vi "Estimate Test Coverage - Main UI - .vi"(10 "Test Path (Tests folder -- including _framework)":path, 11 "Source Path (lvproj, lvclass, vi)":path) -> ()   [LabVIEW 2009]
uses:
  Graphical Test Runner/Graphical Test Runner Support/EstimationResults--Cluster.ctl
  Graphical Test Runner/Graphical Test Runner Support/ScanOptions--Cluster.ctl
  Graphical Test Runner/Graphical Test Runner Support/GraphicalTestRunner.lvlib
panel:
  in  "Estimation Tabs":enum32{"Graphs", "Metrics", "Files", "Setup"}(tab)
  out "Bar Graph":picture caption="Percentage of Test Gaps By Folder"
  in  "Coverage Graph":T1(ring)
  out "Percent Coverage":u8
  out "Total Test VIs":i32
  out "Untested Project VIs":i32
  out "Pass":bool
  in  "Files without coverage":i32(listbox)
  in  "Minimum Coverage (%)":dbl
  in  "Ignore reuse libraries":bool=TRUE
  in  "Ignore non VIs":bool=TRUE
  in  "Abort":bool
  in  "Estimate":bool
  in  "Exit":bool
  # "Estimate Test Coverage"
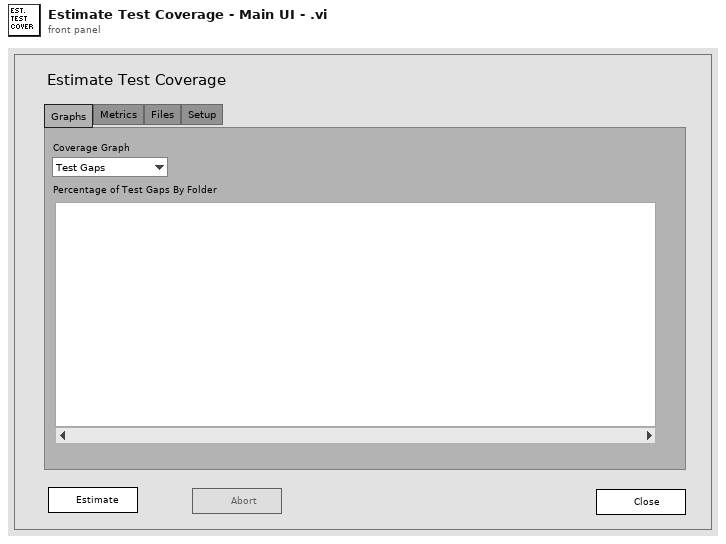
[diagram p1: front panel]
types:
  T1 = enum16{"Test Gaps", "Test Coverage", "Test Failures"}
  T2 = enum32{"Invalid", "Standard", "Closed", "Hidden", "Minimized", "Maximized"}
  T3 = enum32{"invalid app kind", "Development System", "Run Time System", "Student Edition", "Embedded LabVIEW", "Evaluation", "Custom"}
  T4 = typedef "GraphicalTestRunner.lvlib/ScanOptions--Cluster.ctl" = cluster{"Ignore vi.lib":bool, "Ignore user.lib":bool, "Ignore private methods":bool, "Ignore non VIs":bool, "Shallow scan (FALSE)":bool}
  T5 = typedef "GraphicalTestRunner.lvlib/EstimationResults--Cluster.ctl" = cluster{"% Coverage":dbl, "Untested Source VI Count":i32, "Test Hierarchy VI Count":i32}
  T6 = cluster{"Current VI Reference":refnum<vi>, "VIs Without Test Coverage by path":path[], "Coverage Results":T5, "Ignore reuse libraries":bool, "Ignore non VIs":bool}
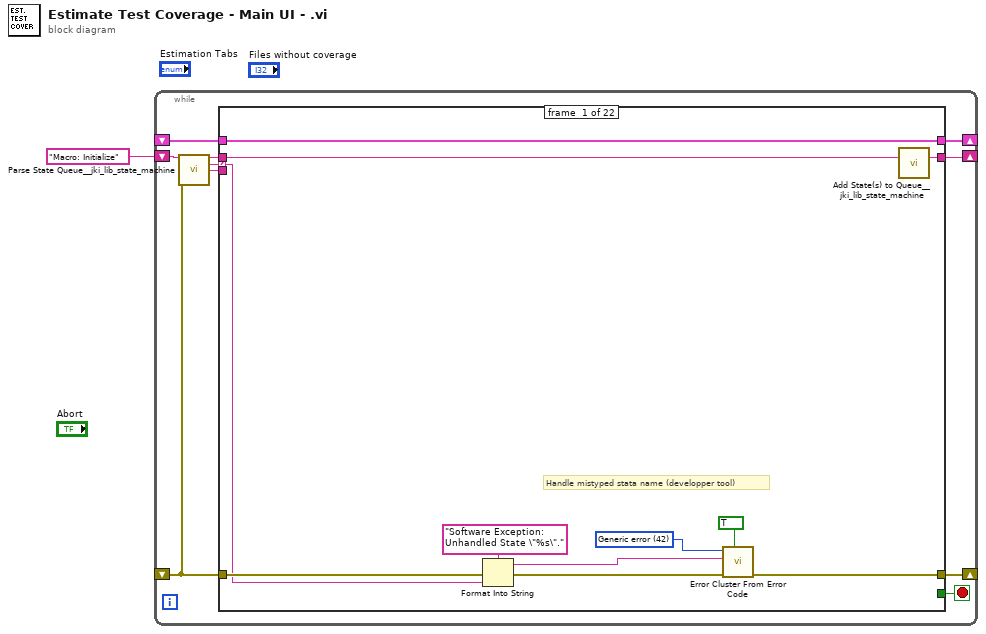
[diagram p0: block diagram]
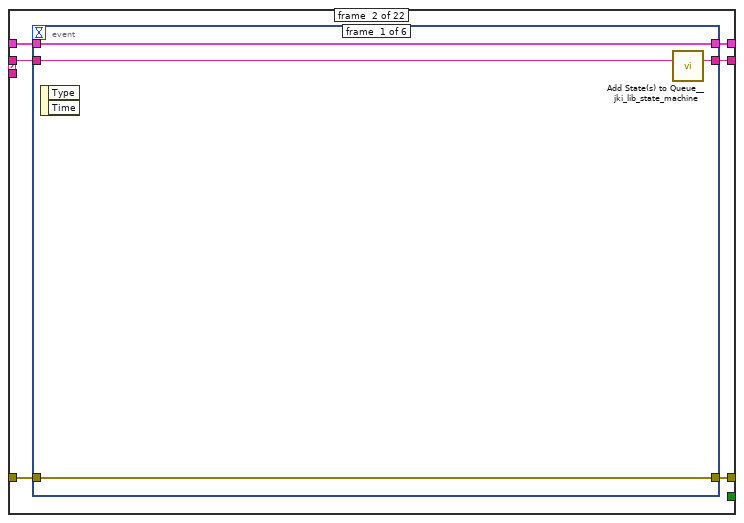
[diagram p2: hidden frame]
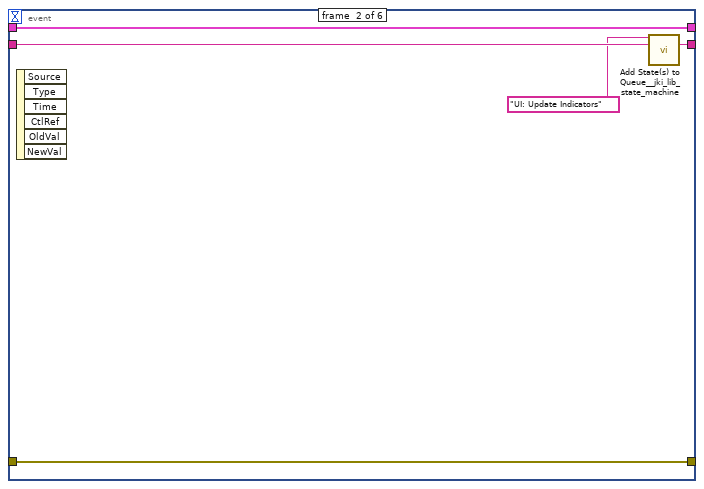
[diagram p3: hidden frame]
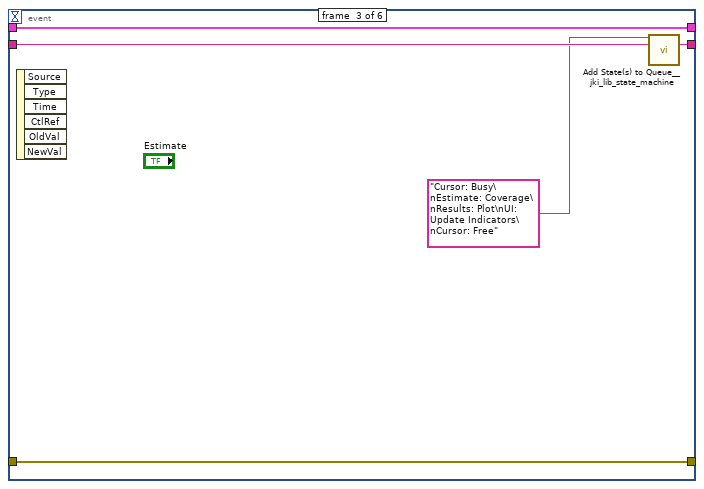
[diagram p4: hidden frame]
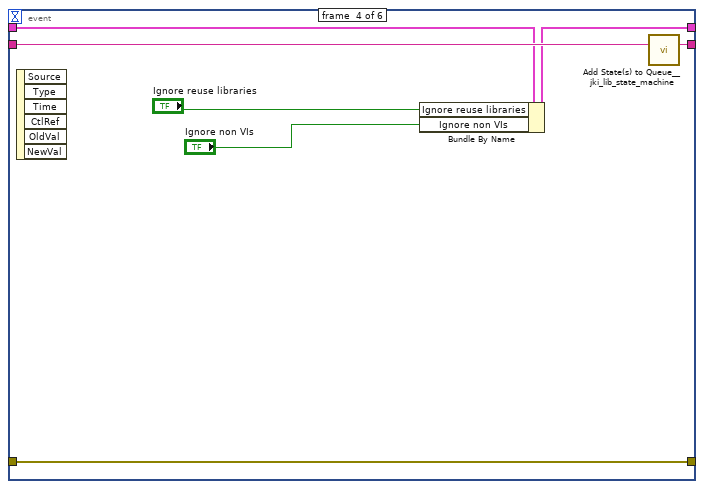
[diagram p5: hidden frame]
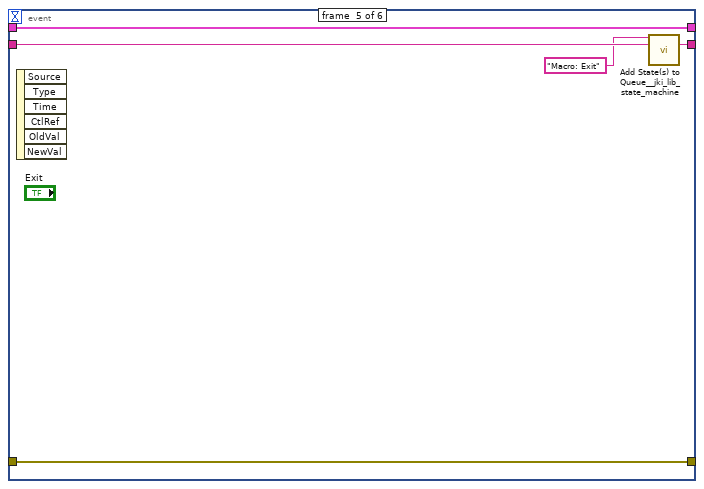
[diagram p6: hidden frame]
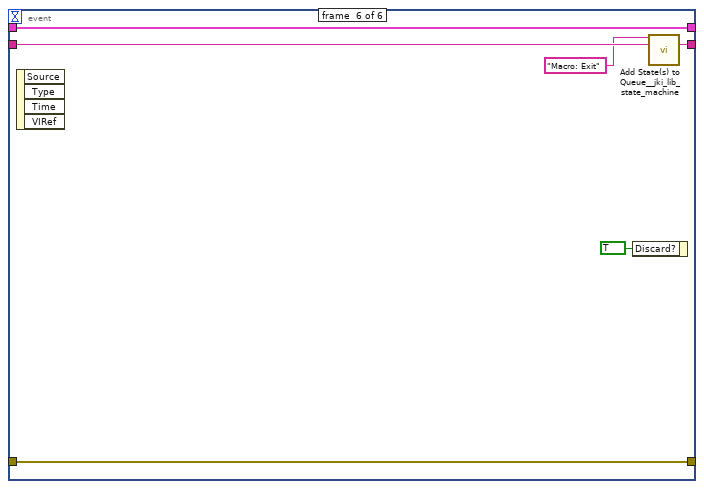
[diagram p7: hidden frame]
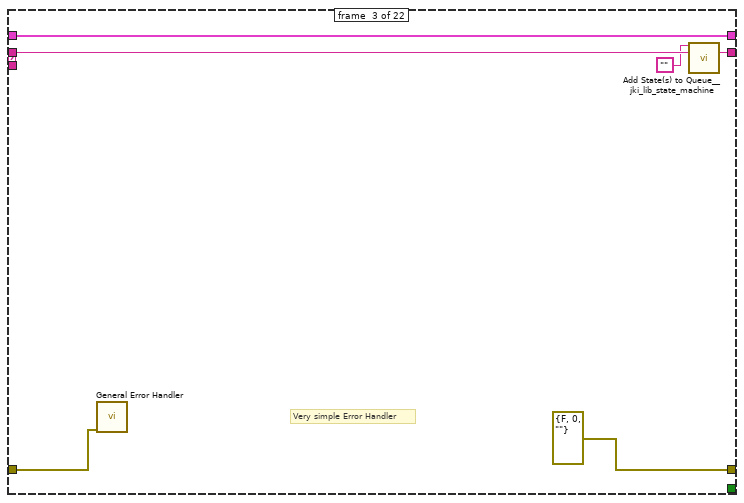
[diagram p8: hidden frame]
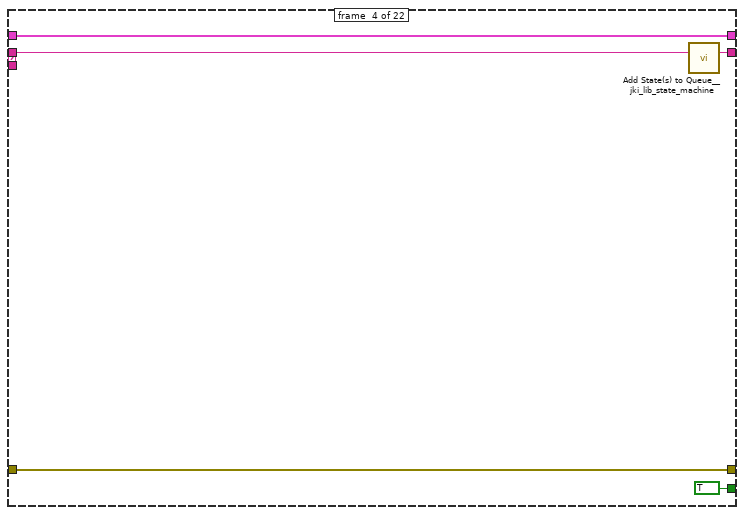
[diagram p9: hidden frame]
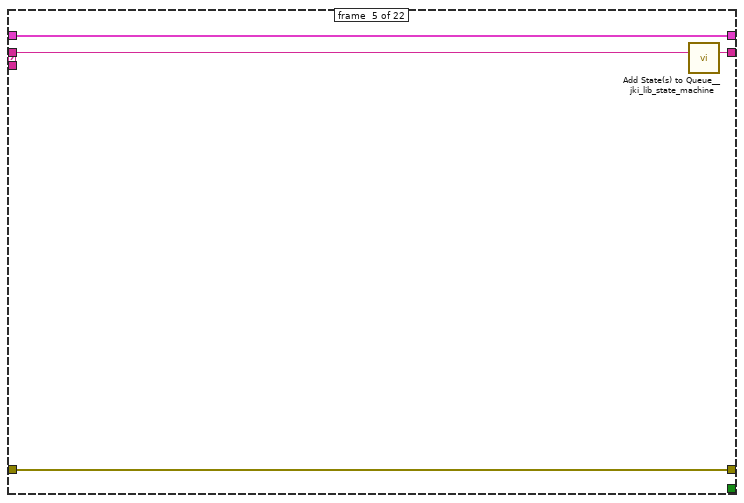
[diagram p10: hidden frame]
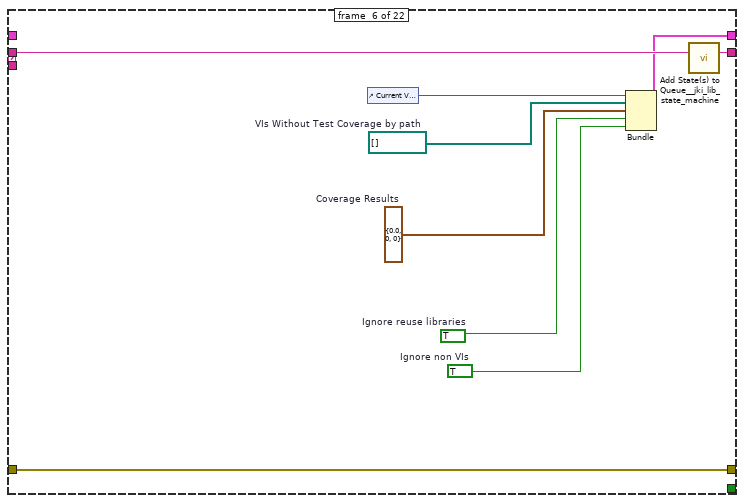
[diagram p11: hidden frame]
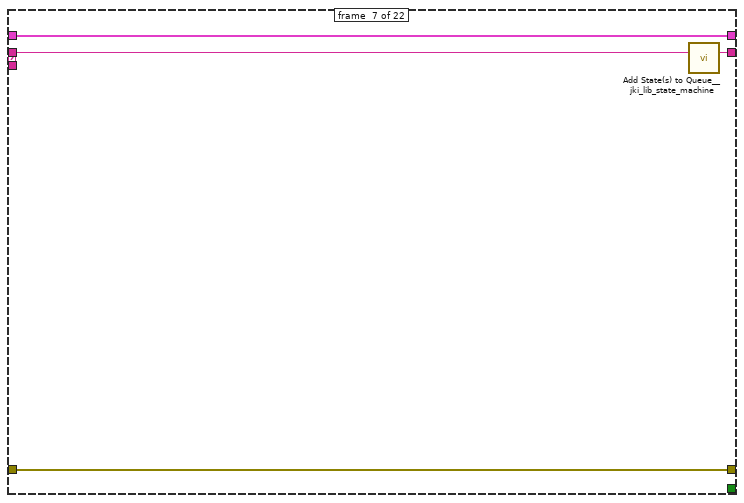
[diagram p12: hidden frame]
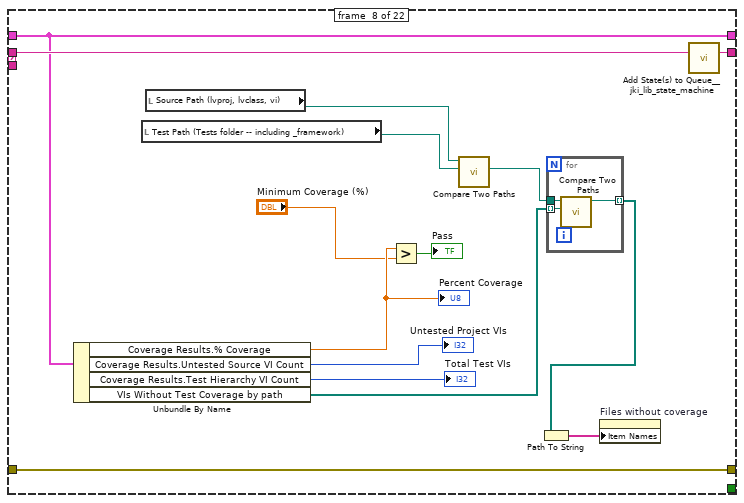
[diagram p13: hidden frame]
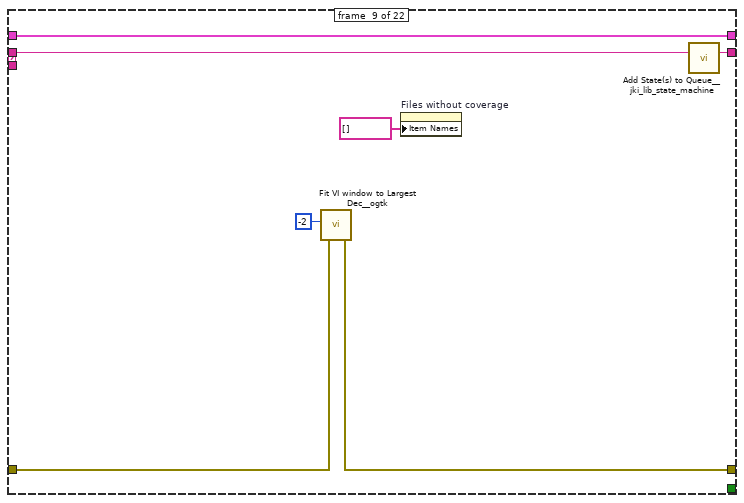
[diagram p14: hidden frame]
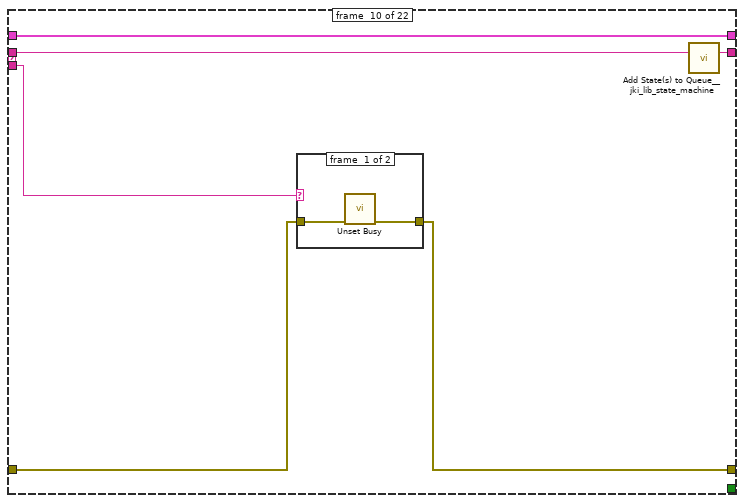
[diagram p15: hidden frame]
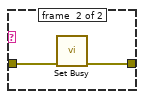
[diagram p16: hidden frame]
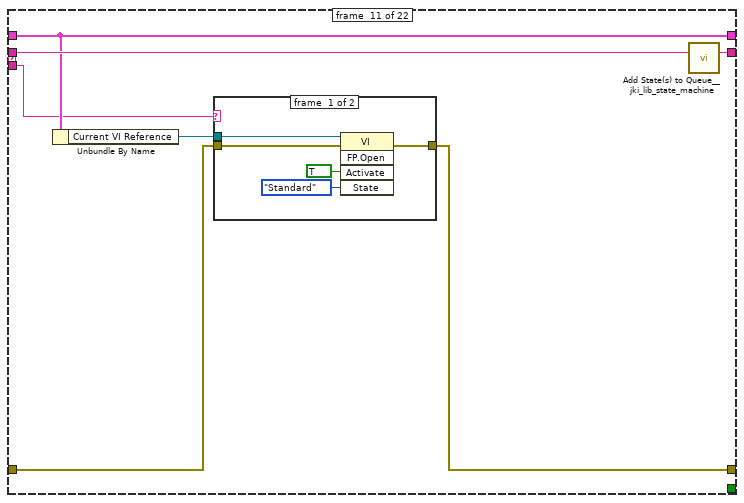
[diagram p17: hidden frame]
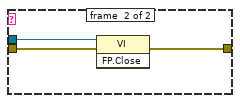
[diagram p18: hidden frame]
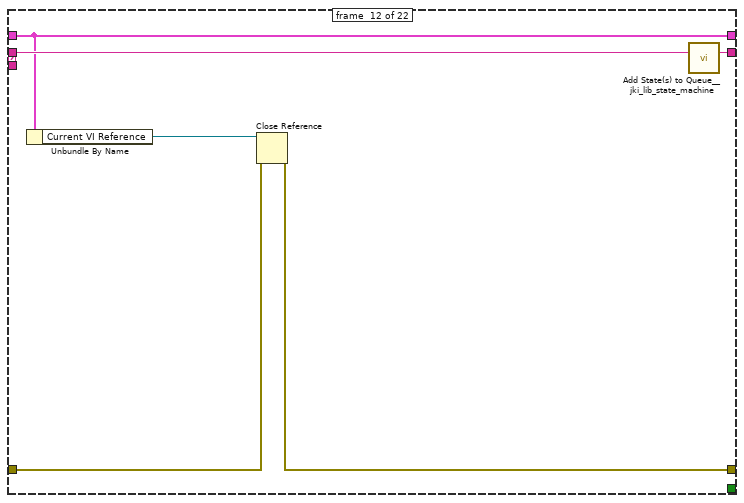
[diagram p19: hidden frame]
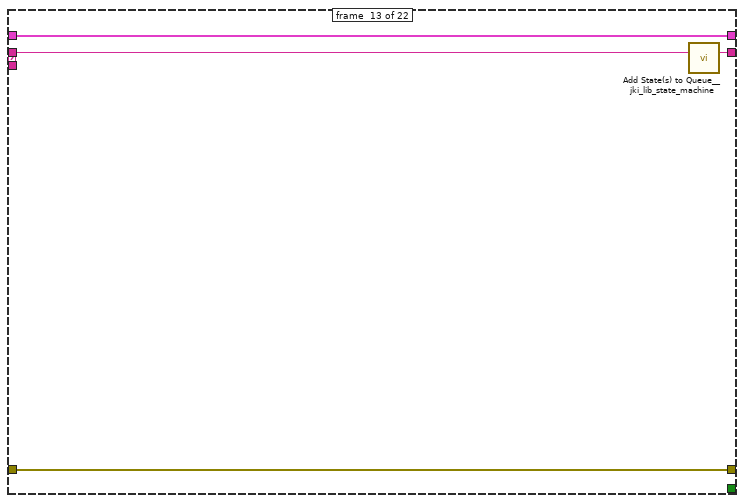
[diagram p20: hidden frame]
diagram:
  n1 = while {
    shift-right: [w2] -> _
    shift-left: _ -> [w7]
    shift-right: [w6] -> _
    shift-left: _ -> [w5]
    shift-right: [w4] -> _
    shift-left: "Macro: Initialize" -> [w8]
    stop <- w3 stop-if-true
    n2 = call <vilib>:"Parse State Queue__jki_lib_state_machine.vi"("State Queue"=w8, "Error In (no error)"=w5) -> ("Remaining States"=w10:string, "Current State"=w11:string, "Arguments"=w9:string)  [unwired: 11 in]
    n3 = case shown="\"Results: Plot\"" w11 {
      selector: w11 -> [w16 _ _ _ _ _ _ _ _ _ _ _ _ _ _ _ _ _ _ _ _ _]
      tunnel: w10 -> [w15 w28 w66 w71 w75 w84 w88 w103 w113 w119 w130 w144 w148 w153 w158 w162 w167 w177 w182 w187 w193 w213]
      tunnel: w9 -> [_ _ _ _ _ _ _ _ _ w114 w126 _ _ _ _ _ _ _ _ _ _ _]
      tunnel: w7 -> [w13 w26 w61 w69 w72 _ w85 w95 w111 w117 w127 w142 w145 w150 w155 w159 w164 w174 w180 w185 w189 w207]
      tunnel: [w18 w25 errorcluster {"status"=FALSE, "code"=0, "source"=""} ("error out") w68 w73 w82 w86 w101 w109 w115 w124 w139 w146 w151 w156 w160 w165 w175 w178 w183 w191 w208] -> w6
      tunnel: w5 -> [w17 w24 w64 w68 w73 w82 w86 w101 w110 w116 w125 w140 w146 w151 w156 w160 w165 w175 w179 w184 w191 w209]
      tunnel: [w14 w27 w65 w70 w74 w83 w87 w102 w112 w118 w129 w143 w147 w152 w157 w161 w166 w176 w181 w186 w192 w212] -> w4
      tunnel: [_ _ _ TRUE _ _ _ _ _ _ _ _ _ _ _ _ _ _ _ _ _ _] -> w3
      tunnel: [w13 w23 w61 w69 w72 w81 w85 w95 w111 w117 w127 w142 w145 w150 w155 w159 w164 w174 w180 w185 w189 w202] -> w2
      frame #0 {
        w21 = 42 items=["No error", "Argument error", "Memory is full", "Out of zone", "End of file", "File already open", "Generic file I/O error", "File not found", "File permission error", "Disk is full", "Duplicate path", "Too many files open", "System feature not enabled", "Resource file not found", "Cannot add resource", "Resource not found", "Image not found", "Image memory error", "Pen does not exist", "Config type invalid", "Config token not found", "Config parse error", "Config memory error", "Bad external code format", "Bad external code offset", "External code not present", "Null window", "Destroy window error", "Null menu", "Print aborted", "Bad print record", "Print driver error", "Windows error during printing", "Memory error during printing", "Print dialog error", "Generic print error", "Invalid device refnum", "Device not found", "Device parameter error", "Device unit error", "Cannot open device", "Device call aborted", "Generic error", "Cancelled by user", "Object ID too low", "Object ID too high", "Object not in heap", "Unknown heap", "Unknown object (invalid DefProc)", "Unknown object (DefProc not in table)", "Message out of range", "Invalid (null) method", "Unknown message", "Manager call not supported", "Bad address", "Network operation in progress", "Network operation timed out", "Connection is busy", "Network attribute not supported", "Network error", "Address in use", "System out of memory", "Connection aborted", "Connection refused", "Not connected", "Already connected", "Connection closed", "Initialization error (interapplication manager)", "Bad occurrence", "Wait on unbound occurrence handler", "Occurrence queue overflow", "Datalog type conflict", "Unused", "Unrecognized type (interapplication manager)", "Memory corrupt", "Failed to make temporary DLL", "Old CIN version", "Drag socket not found", "Failed to load drop-object", "Failed to register OLE object", "Failed to release OLE object", "Format specifier type mismatch", "Unknown format specifier", "Too few format specifiers", "Too many format specifiers", "Scan failed", "Newer CIN version", "Error converting to variant", "Runtime menu error", "Password tampered", "Variant attribute not found", "Incompatible variant data type", "Event data is not available", "Event Store is not present", "Occurrence is not found", "Event Queue is not created", "Event info is not available", "Refnum passed is NULL", "Error retrieving Class GUID", "Error retrieving CoClass GUID", "Error retrieving TypeLib GUID.", "Bad built application magic bytes.", "Specific driver is different from the specific driver associated with the Logical Name.", "There is no session opened to the class driver.", "Max Error", "MAX - Error with config objects", "MAX - Error loading configuration", "MAX - Group not supported"]
        # "Handle mistyped stata name (developper tool)"
        n4 = Format Into String(format string="Software Exception: Unhandled State \"%s\"." ("message"), error in=w17, w16) -> (resulting string=w20:string, error out=w19:errorcluster)  [unwired: 1 in]
        n5 = call <vilib>:"Error Cluster From Error Code.vi"("show call chain? (False)"=TRUE, "error in (no error)"=w19, "error message (\"\")"=w20, "error code (0)"=w21) -> ("error out"=w18:errorcluster)  [unwired: 5 in]
        n6 = call <vilib>:"Add State(s) to Queue__jki_lib_state_machine.vi"("State(s) in (\"\")"=w15) -> ("States Out"=w14:string)  [unwired: 14 in]
      }
      frame #1 {
        n7 = event shown="[2] \"Estimate\": Value Change" {
          selector: _ -> [_ _ _ _ _ _]
          dyn-events: _ -> [_ _ _ _ _ _]
          timeout: _ -> [_ _ _ _ _ _]
          tunnel: w28 -> [w32 w37 w42 w49 w54 w60]
          tunnel: [w31 w36 w41 w48 w53 w59] -> w27
          tunnel: w26 -> [w29 w34 w39 w46 w51 w57]
          tunnel: [w30 w35 w40 w47 w52 w58] -> w25
          tunnel: w24 -> [w30 w35 w40 w47 w52 w58]
          tunnel: [w29 w34 w39 w45 w51 w57] -> w23
          event #0 {
            n8 = event-data() -> ()  [unwired: 1 in, 2 out]
            n9 = call <vilib>:"Add State(s) to Queue__jki_lib_state_machine.vi"("State(s) in (\"\")"=w32) -> ("States Out"=w31:string)  [unwired: 14 in]
          }
          event #1 {
            n10 = event-data() -> ()  [unwired: 1 in, 6 out]
            n11 = call <vilib>:"Add State(s) to Queue__jki_lib_state_machine.vi"("State(s) in Front (\"\")"="UI: Update Indicators" ("State(s) in Front"), "State(s) in (\"\")"=w37) -> ("States Out"=w36:string)  [unwired: 13 in]
          }
          event #2 {
            n12 = event-data() -> ()  [unwired: 1 in, 6 out]
            n13 = call <vilib>:"Add State(s) to Queue__jki_lib_state_machine.vi"("State(s) in Front (\"\")"="Cursor: Busy\nEstimate: Coverage\nResults: Plot\nUI: Update Indicators\nCursor: Free" ("State(s) in Front"), "State(s) in (\"\")"=w42) -> ("States Out"=w41:string)  [unwired: 13 in]
          }
          event #3 {
            n14 = event-data() -> ()  [unwired: 1 in, 6 out]
            n15 = Bundle By Name(cluster=w46, "Ignore reuse libraries"="Ignore reuse libraries", "Ignore non VIs"="Ignore non VIs") -> (w45:T6)
            n16 = call <vilib>:"Add State(s) to Queue__jki_lib_state_machine.vi"("State(s) in (\"\")"=w49) -> ("States Out"=w48:string)  [unwired: 14 in]
          }
          event #4 {
            n17 = event-data() -> ()  [unwired: 1 in, 6 out]
            n18 = call <vilib>:"Add State(s) to Queue__jki_lib_state_machine.vi"("State(s) in Front (\"\")"="Macro: Exit", "State(s) in (\"\")"=w54) -> ("States Out"=w53:string)  [unwired: 13 in]
          }
          event #5 {
            n19 = event-data() -> ()  [unwired: 1 in, 4 out]
            n20 = event-data("Discard?"=TRUE) -> ()  [unwired: 1 in, 1 out]
            n21 = call <vilib>:"Add State(s) to Queue__jki_lib_state_machine.vi"("State(s) in Front (\"\")"="Macro: Exit", "State(s) in (\"\")"=w60) -> ("States Out"=w59:string)  [unwired: 13 in]
          }
        }
      }
      frame #2 {
        # "Very simple Error Handler"
        n22 = call <vilib>:"General Error Handler.vi"("error in (no error)"=w64) -> ()  [unwired: 10 in, 5 out]
        n23 = call <vilib>:"Add State(s) to Queue__jki_lib_state_machine.vi"("State(s) in Front (\"\")"="", "State(s) in (\"\")"=w66) -> ("States Out"=w65:string)  [unwired: 13 in]
      }
      frame #3 {
        n24 = call <vilib>:"Add State(s) to Queue__jki_lib_state_machine.vi"("State(s) in (\"\")"=w71) -> ("States Out"=w70:string)  [unwired: 14 in]
      }
      frame #4 {
        n25 = call <vilib>:"Add State(s) to Queue__jki_lib_state_machine.vi"("State(s) in (\"\")"=w75) -> ("States Out"=w74:string)  [unwired: 14 in]
      }
      frame #5 {
        w76 = TRUE  # Ignore non VIs
        w77 = TRUE  # Ignore reuse libraries
        w78 = T5 {"% Coverage"=0.0, "Untested Source VI Count"=0, "Test Hierarchy VI Count"=0}  # Coverage Results
        w79 = path[] []  # VIs Without Test Coverage by path
        n26 = control-ref of="Current VI Reference"() -> (w80:refnum<vi>)
        n27 = Bundle("Current VI Reference"=w80, "VIs Without Test Coverage by path"=w79, "Coverage Results"=w78, "Ignore reuse libraries"=w77, "Ignore non VIs"=w76) -> (w81:T6)  [unwired: 1 in]
        n28 = call <vilib>:"Add State(s) to Queue__jki_lib_state_machine.vi"("State(s) in (\"\")"=w84) -> ("States Out"=w83:string)  [unwired: 14 in]
      }
      frame #6 {
        n29 = call <vilib>:"Add State(s) to Queue__jki_lib_state_machine.vi"("State(s) in (\"\")"=w88) -> ("States Out"=w87:string)  [unwired: 14 in]
      }
      frame #7 {
        n30 = Unbundle By Name(w95) -> ("Coverage Results.% Coverage"=w98:dbl, "Coverage Results.Untested Source VI Count"=→"Untested Project VIs":i32, "Coverage Results.Test Hierarchy VI Count"=→"Total Test VIs":i32, "VIs Without Test Coverage by path"=w90:path[])
        "Percent Coverage" <- w98
        n31 = local read "Test Path (Tests folder -- including _framework)"() -> (w92:path)
        n32 = local read "Source Path (lvproj, lvclass, vi)"() -> (w93:path)
        n33 = Greater?(x=w98, y="Minimum Coverage (%)") -> (0:→"Pass":bool)
        n34 = call <vilib>:"Compare Two Paths.vi"("Path 2"=w92, "Path 1"=w93) -> ("Common Path"=w91:path)  [unwired: 6 in, 3 out]
        n35 = for {
          tunnel: w91 -> [w106]
          tunnel: w90 -> [w105] mode=indexing
          tunnel: [w104] -> w89 mode=indexing
          n36 = call <vilib>:"Compare Two Paths.vi"("Path 2"=w105, "Path 1"=w106) -> ("Relative Path from 1 to 2"=w104:path)  [unwired: 6 in, 3 out]
        }
        n37 = Path To String(path=w89) -> (string=w94:string[])
        n38 = property on="Files without coverage" class="LstBox (strict)"("Item Names"=w94) -> ()  [unwired: 2 in, 2 out]
        n39 = call <vilib>:"Add State(s) to Queue__jki_lib_state_machine.vi"("State(s) in (\"\")"=w103) -> ("States Out"=w102:string)  [unwired: 14 in]
      }
      frame #8 {
        n40 = call <userlib>:"Fit VI window to Largest Dec__ogtk.vi"("error in (no error)"=w110, "border spacing (2 px)"=-2) -> ("error out"=w109:errorcluster)  [unwired: 4 in, 1 out]
        n41 = property on="Files without coverage" class="LstBox (strict)"("Item Names"=string[] []) -> ()  [unwired: 2 in, 2 out]
        n42 = call <vilib>:"Add State(s) to Queue__jki_lib_state_machine.vi"("State(s) in (\"\")"=w113) -> ("States Out"=w112:string)  [unwired: 14 in]
      }
      frame #9 {
        n43 = case shown="\"Idle\", Default" w114 {
          tunnel: w116 -> [w121 w123]
          tunnel: [w120 w122] -> w115
          frame #0 {
            n44 = call <vilib>:"Unset Busy.vi"("error in (no error)"=w121) -> ("error out"=w120:errorcluster)  [unwired: 10 in]
          }
          frame #1 {
            n45 = call <vilib>:"Set Busy.vi"("error in (no error)"=w123) -> ("error out"=w122:errorcluster)  [unwired: 9 in, 1 out]
          }
        }
        n46 = call <vilib>:"Add State(s) to Queue__jki_lib_state_machine.vi"("State(s) in (\"\")"=w119) -> ("States Out"=w118:string)  [unwired: 14 in]
      }
      frame #10 {
        n47 = Unbundle By Name(w127) -> ("Current VI Reference"=w128:refnum<vi>)
        n48 = case shown="\"Close\"" w126 {
          tunnel: w128 -> [w133 w138]
          tunnel: w125 -> [w132 w137]
          tunnel: [w131 w136] -> w124
          frame #0 {
            n49 = invoke class="VI" method="FP.Open"(reference=w133, error in=w132, "Activate"=TRUE, "State"=T2."Standard") -> (error out=w131:errorcluster)  [unwired: 1 in, 4 out]
          }
          frame #1 {
            n50 = invoke class="VI" method="FP.Close"(reference=w138, error in=w137) -> (error out=w136:errorcluster)  [unwired: 1 in, 2 out]
          }
        }
        n51 = call <vilib>:"Add State(s) to Queue__jki_lib_state_machine.vi"("State(s) in (\"\")"=w130) -> ("States Out"=w129:string)  [unwired: 14 in]
      }
      frame #11 {
        n52 = Unbundle By Name(w142) -> ("Current VI Reference"=w141:refnum<vi>)
        n53 = Close Reference(reference=w141, error in (no error)=w140) -> (error out=w139:errorcluster)
        n54 = call <vilib>:"Add State(s) to Queue__jki_lib_state_machine.vi"("State(s) in (\"\")"=w144) -> ("States Out"=w143:string)  [unwired: 14 in]
      }
      frame #12 {
        n55 = call <vilib>:"Add State(s) to Queue__jki_lib_state_machine.vi"("State(s) in (\"\")"=w148) -> ("States Out"=w147:string)  [unwired: 14 in]
      }
      frame #13 {
        w149 = "App Data: Initialize\nUI: Initialize\nUI: Front Panel State >> Open"  # App Data: Initialize UI: Initialize UI: Front Panel State >> Open
        n56 = call <vilib>:"Add State(s) to Queue__jki_lib_state_machine.vi"("State(s) in Front (\"\")"=w149, "State(s) in (\"\")"=w153) -> ("States Out"=w152:string)  [unwired: 13 in]
      }
      frame #14 {
        n57 = call <vilib>:"Add State(s) to Queue__jki_lib_state_machine.vi"("State(s) in Front (\"\")"="/*Condition: Check for Panel Close at Exit\nUI: Front Panel State >> Close\nUI: References Cleanup\nExit", "State(s) in (\"\")"=w158) -> ("States Out"=w157:string)  [unwired: 13 in]
      }
      frame #15 {
        n58 = call <vilib>:"Add State(s) to Queue__jki_lib_state_machine.vi"("State(s) in (\"\")"=w162) -> ("States Out"=w161:string)  [unwired: 14 in]
      }
      frame #16 {
        n59 = stacked-sequence {
          tunnel: [w173] -> w163
          frame #0 {
            n60 = property class="App"() -> ("App.Kind"=w170:T3)  [unwired: 2 in, 2 out]
            n61 = Equal?(x=w170, y=T3."Development System") -> (x = y?=w169:bool)
            n62 = Select(t="", s=w169, f="UI: Front Panel State >> Close") -> (s? t:f=w173:string)
          }
        }
        n63 = call <vilib>:"Add State(s) to Queue__jki_lib_state_machine.vi"("State(s) in Front (\"\")"=w163, "State(s) in (\"\")"=w167) -> ("States Out"=w166:string)  [unwired: 13 in]
      }
      frame #17 {
        n64 = call <vilib>:"Add State(s) to Queue__jki_lib_state_machine.vi"("State(s) in (\"\")"=w177) -> ("States Out"=w176:string)  [unwired: 14 in]
      }
      frame #18 {
        n65 = call <vilib>:"Set Busy.vi"("error in (no error)"=w179) -> ("error out"=w178:errorcluster)  [unwired: 9 in, 1 out]
        n66 = call <vilib>:"Add State(s) to Queue__jki_lib_state_machine.vi"("State(s) in (\"\")"=w182) -> ("States Out"=w181:string)  [unwired: 14 in]
      }
      frame #19 {
        n67 = call <vilib>:"Unset Busy.vi"("error in (no error)"=w184) -> ("error out"=w183:errorcluster)  [unwired: 10 in]
        n68 = call <vilib>:"Add State(s) to Queue__jki_lib_state_machine.vi"("State(s) in (\"\")"=w187) -> ("States Out"=w186:string)  [unwired: 14 in]
      }
      frame #20 {
        n69 = Unbundle By Name(w189) -> ("VIs Without Test Coverage by path"=w188:path[])
        n70 = case shown="\"Test Gaps\", Default" "Coverage Graph" {
          tunnel: w188 -> [w199]
          frame "Test Gaps", Default {
            (unwired) u32[] [6618880, 16773465, 16711680, 393471, 16758082, 14559999, 10551291] ("colors")
            n71 = call "Calculate Test Gaps.vi"("VIs Without Test Coverage by path"=w199) -> ("folder names"=w197:string[], "% of gap values"=w198:dbl[])  [unwired: 9 in]
            n72 = Build Array(u32 393471 ("color(black)")) -> (w194:u32[])
            n73 = call "Create Bar Graph.vi"("colors"=w194, "names"=w197, "values"=w198) -> ("Bar Graph"=→"Bar Graph":picture)  [unwired: 8 in]
          }
        }
        n74 = call <vilib>:"Add State(s) to Queue__jki_lib_state_machine.vi"("State(s) in (\"\")"=w193) -> ("States Out"=w192:string)  [unwired: 14 in]
      }
      frame #21 {
        n75 = Unbundle By Name(w207) -> ("Ignore reuse libraries"=w204:bool, "Ignore non VIs"=w203:bool)
        n76 = Bundle By Name(cluster=T4 {"Ignore vi.lib"=TRUE, "Ignore user.lib"=TRUE, "Ignore private methods"=TRUE, "Ignore non VIs"=TRUE, "Shallow scan (FALSE)"=FALSE} ("Scan Options"), "Ignore vi.lib"=w204, "Ignore user.lib"=w204, "Ignore non VIs"=w203) -> (w205:T4)
        n77 = call "Estimate Test Coverage.vi"("error in (no error)"=w209, "Scan Options"=w205, "Test Path (Tests folder -- including _framework)"="Test Path (Tests folder -- including _framework)", "Source Path (lvproj, lvclass, vi)"="Source Path (lvproj, lvclass, vi)") -> ("error out"=w208:errorcluster, "Coverage Results"=w200:T5, "VIs Without Test Coverage by path"=w201:path[])  [unwired: 5 in]
        n78 = Bundle By Name(cluster=w207, "VIs Without Test Coverage by path"=w201, "Coverage Results"=w200) -> (w202:T6)
        n79 = call <vilib>:"Add State(s) to Queue__jki_lib_state_machine.vi"("State(s) in (\"\")"=w213) -> ("States Out"=w212:string)  [unwired: 14 in]
      }
    }
  }
